vi "(SubVI)Calculate zbd for Wang97 .vi"(0 "ztrap (nm)":dbl=300.0, 2 "kxz":dbl=3.6) -> (7 "Zbd":dbl)   [LabVIEW 2014]
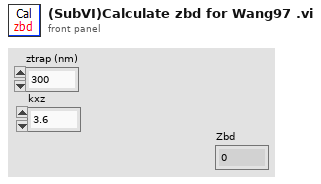
[diagram p1: front panel]
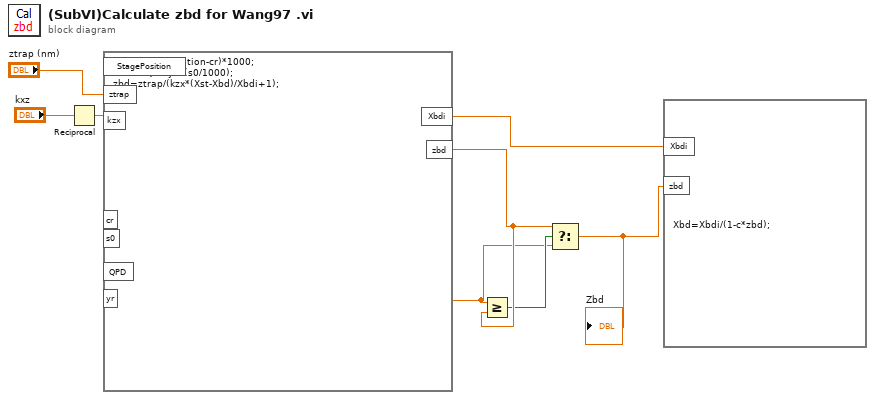
[diagram p0: block diagram]
diagram:
  n1 = Reciprocal(x="kxz") -> (1/x=w6:dbl)
  n2 = formula code="Xst=(StagePosition-cr)*1000;\nXbdi=(QPD-yr)/(s0/1000);\nzbd=ztrap/(kzx*(Xst-Xbd)/Xbdi+1);"("ztrap"="ztrap (nm)", "kzx"=w6) -> ("zbd"=w5:dbl, "Xbdi"=w2:dbl)  [unwired: 5 in]
  n3 = Greater Or Equal?(x="ztrap (nm)", y=w5) -> (x >= y?=w4:bool)
  n4 = Select(t=w5, s=w4, f="ztrap (nm)") -> (s? t:f=w1:dbl)
  "Zbd" <- w1
  n5 = formula code="Xbd=Xbdi/(1-c*zbd);"("Xbdi"=w2, "zbd"=w1) -> ()
